vi "Get Generation Status and Type.vi"(8 "error in (no error)":errorcluster) -> (0 "error out":errorcluster, 3 "type and status":T1)   [LabVIEW 2021, in "AudioGenTCPReaderProcess.lvlib"]
uses:
  AudioGenTCPReaderProcess.lvlib
  controls/generation status.ctl
  controls/AudioGenTypeDefs.lvlib
  controls/generation type.ctl
  controls/generation type and status.ctl
  Digital Audio Generation/DigitalAudioGenerationProcess.lvlib
  Analog Generation/AnalogGenerationProcess.lvlib
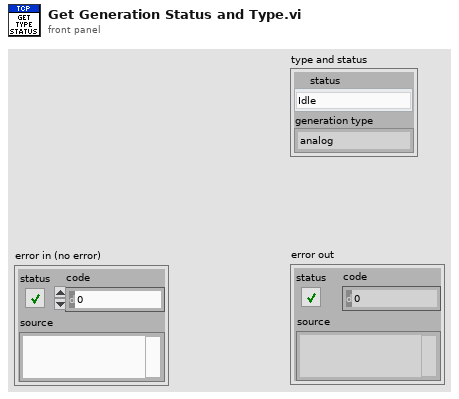
[diagram p1: front panel]
types:
  T1 = typedef "AudioGenTypeDefs.lvlib/generation type and status.ctl" = cluster{"status":T2, "generation type":T3}
  T2 = typedef "AudioGenTypeDefs.lvlib/generation status.ctl" = enum16{"Idle", "Committed", "Active"}
  T3 = typedef "AudioGenTypeDefs.lvlib/generation type.ctl" = enum16{"analog", "digital"}
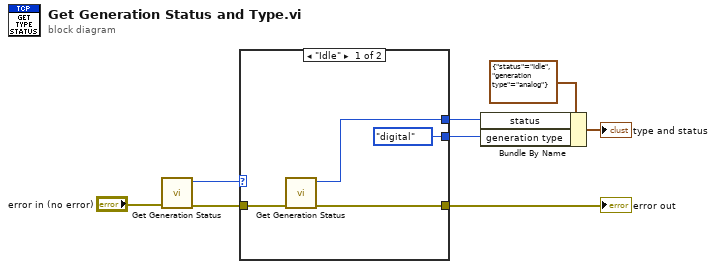
[diagram p0: block diagram]
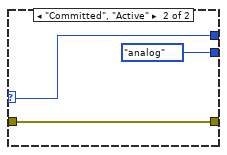
[diagram p2: hidden frame]
diagram:
  n1 = call "Get Generation Status.vi"("error in (no error)"="error in (no error)") -> ("error out"=w4:errorcluster, "generation status"=w5:T2)  [unwired: 9 in]
  n2 = case shown="\"Idle\"" w5 {
    selector: w5 -> [_ w14]
    tunnel: w4 -> [w12 w13]
    tunnel: [w11 w14] -> w3
    tunnel: [generation_type."digital" ("generation type") generation_type."analog" ("generation type")] -> w2
    tunnel: [w9 w13] -> w1
    frame "Idle" {
      n3 = call "Get Generation Status.vi"("error in (no error)"=w12) -> ("error out"=w9:errorcluster, "generation status"=w11:T2)  [unwired: 9 in]
    }
    frame "Committed", "Active" {
    }
  }
  "error out" <- w1
  n4 = Bundle By Name(cluster=T1 {"status"=enum."Idle", "generation type"=enum."analog"} ("generation"), "status"=w3, "generation type"=w2) -> (→"type and status":T1)
